vi "Close.vi"(8 "Error In":errorcluster, 11 "Open Weather Session In":refnum<class "Open Weather Session.lvclass">) -> (0 "Error Out":errorcluster)   [LabVIEW 2019, in "Open Weather Session.lvclass"]
uses:
  Open Weather Session.lvclass
  Accessors/REST Client/Get REST Client.vi
  <vilib>/addons/_JKI.lib/REST Client/classes/REST Client/REST Client.lvclass
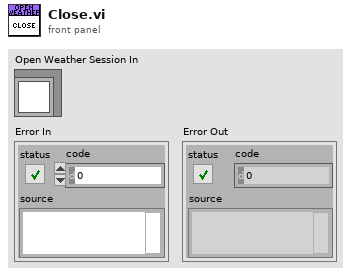
[diagram p1: front panel]
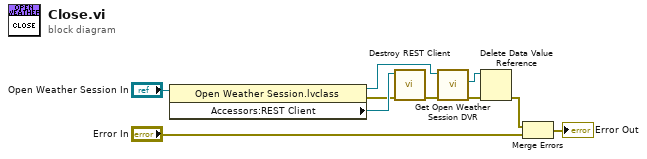
[diagram p0: block diagram]
diagram:
  n1 = property class="Open Weather Session.lvclass"(reference="Open Weather Session In") -> (reference out=w4:refnum<class "Open Weather Session.lvclass">, error out=w8:errorcluster, "Accessors:REST Client"=w9:refnum<class "REST Client.lvclass">)  [unwired: 1 in]
  n2 = call-dynamic "Destroy REST Client.vi"("error in (no error)"=w8, "REST Client in"=w9) -> ("error out"=w5:errorcluster)  [unwired: 9 in]
  n3 = call "Get Open Weather Session DVR.vi"("Error In"=w5, "Open Weather Session In"=w4) -> ("Error Out"=w3:errorcluster, "DVR"=w2:refnum<data-value>)  [unwired: 7 in, 1 out]
  n4 = Delete Data Value Reference(data value reference=w2, error in=w3) -> (error out=w1:errorcluster)  [unwired: 1 out]
  n5 = Merge Errors(w1, "Error In") -> (→"Error Out":errorcluster)
